vi "Open_WeatherStation_Connection.vi"(1 "Station ID":i32, 2 "Baud rate":i32, 3 "COM port":i32) -> (0 "Weather station connected?":bool)   [LabVIEW 2013]
uses:
  Globals/USB_WeatherLink_Serialnumber.vi
  VantagePro.dll
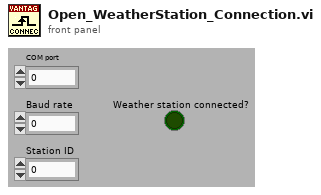
[diagram p1: front panel]
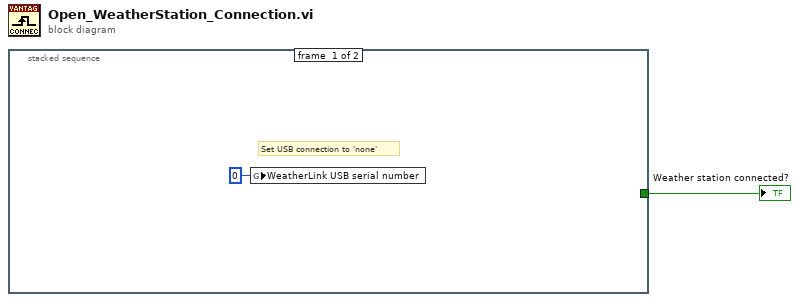
[diagram p0: block diagram]
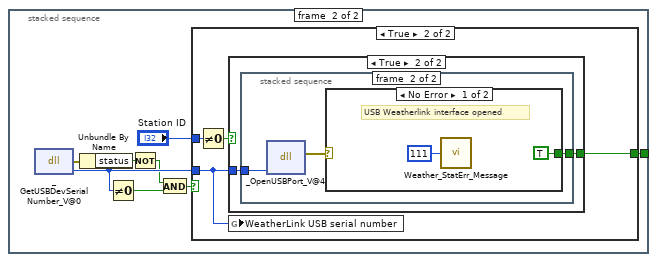
[diagram p2: hidden frame]
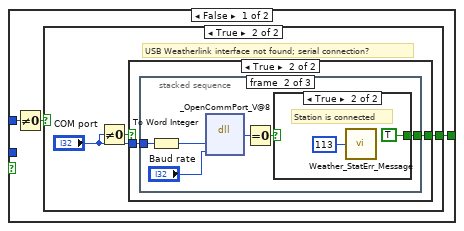
[diagram p3: hidden frame]
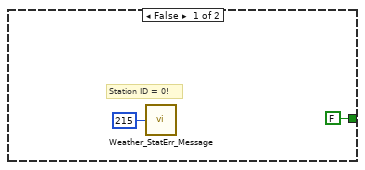
[diagram p4: hidden frame]
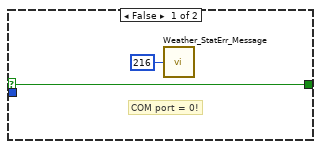
[diagram p5: hidden frame]
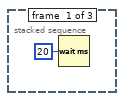
[diagram p6: hidden frame]
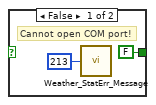
[diagram p7: hidden frame]
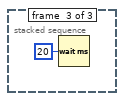
[diagram p8: hidden frame]
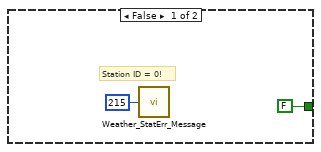
[diagram p9: hidden frame]
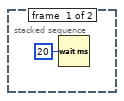
[diagram p10: hidden frame]
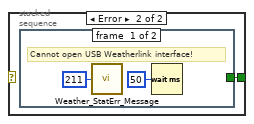
[diagram p11: hidden frame]
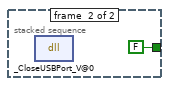
[diagram p12: hidden frame]
diagram:
  n1 = stacked-sequence {
    tunnel: [_ w3] -> w1
    frame #0 {
      # "Set USB connection to 'none'"
      n2 = global write "USB_WeatherLink_Serialnumber.vi" "WeatherLink USB serial number"(u32 0 ("WeatherLink USB serial number")) -> ()
    }
    frame #1 {
      n3 = dll-call lib="C:/Users/Bob van Eijk/Desktop/LabView Projects 13/HiSPARC Weather Station/Develop/VantagePro.dll" fn="_GetUSBDevSerialNumber_V@0" label="Get USB Device\nSerial Number"() -> (error out=w9:errorcluster, "return type"=w8:u32)  [unwired: 3 in, 1 out]
      n4 = Unbundle By Name(w9) -> ("status"=w6:bool)
      n5 = Not Equal To 0?(x=w8) -> (x != 0?=w7:bool)
      n6 = Not(x=w6) -> (.not. x?=w5:bool)
      n7 = And(x=w5, y=w7) -> (x .and. y?=w10:bool)
      n8 = case shown="True" w10 {
        tunnel: [w13 w38] -> w3
        tunnel: w8 -> [_ w35]
        tunnel: "Station ID" -> [w12 w37]
        frame False {
          n9 = Not Equal To 0?(x=w12) -> (x != 0?=w11:bool)
          n10 = case shown="True" w11 {
            tunnel: [FALSE w16] -> w13
            frame False {
              # "Station ID = 0!"
              n11 = call "Weather_StatErr_Message.vi"("Message number"=215) -> ()  [unwired: 1 out]
            }
            frame True {
              # "USB Weatherlink interface not found; serial connection?"
              n12 = Not Equal To 0?(x="COM port") -> (x != 0?=w18:bool)
              n13 = case shown="True" w18 {
                selector: w18 -> [w20 _]
                tunnel: "COM port" -> [_ w22]
                tunnel: [w20 w21] -> w16
                frame False {
                  # "COM port = 0!"
                  n14 = call "Weather_StatErr_Message.vi"("Message number"=216) -> ()  [unwired: 1 out]
                }
                frame True {
                  n15 = stacked-sequence {
                    tunnel: w22 -> [_ w28 _]
                    tunnel: [_ w24 _] -> w21
                    frame #0 {
                      n16 = Wait (ms)(milliseconds to wait=u32 20) -> ()  [unwired: 1 out]
                    }
                    frame #1 {
                      n17 = To Word Integer(number=w28) -> (16bit integer=w27:i16)
                      n18 = dll-call lib="C:/Users/Bob van Eijk/Desktop/LabView Projects 13/HiSPARC Weather Station/Develop/VantagePro.dll" fn="_OpenCommPort_V@8" label="OpenCommPort_V"("comPort"=w27, "baudRate"="Baud rate") -> ("return type"=w26:i16)  [unwired: 4 in, 3 out]
                      n19 = Equal To 0?(x=w26) -> (x = 0?=w25:bool)
                      n20 = case shown="True" w25 {
                        tunnel: [FALSE TRUE] -> w24
                        frame False {
                          # "Cannot open COM port!"
                          n21 = call "Weather_StatErr_Message.vi"("Message number"=213) -> ()  [unwired: 1 out]
                        }
                        frame True {
                          # "Station is connected"
                          n22 = call "Weather_StatErr_Message.vi"("Message number"=113) -> ()  [unwired: 1 out]
                        }
                      }
                    }
                    frame #2 {
                      n23 = Wait (ms)(milliseconds to wait=u32 20) -> ()  [unwired: 1 out]
                    }
                  }
                }
              }
            }
          }
        }
        frame True {
          n24 = Not Equal To 0?(x=w37) -> (x != 0?=w36:bool)
          n25 = case shown="True" w36 {
            tunnel: [FALSE ("USB interface?") w42] -> w38
            tunnel: w35 -> [_ w41]
            frame False {
              # "Station ID = 0!"
              n26 = call "Weather_StatErr_Message.vi"("Message number"=215) -> ()  [unwired: 1 out]
            }
            frame True {
              n27 = stacked-sequence {
                tunnel: [_ w46] -> w42
                tunnel: w41 -> [_ w45]
                frame #0 {
                  n28 = Wait (ms)(milliseconds to wait=u32 20) -> ()  [unwired: 1 out]
                }
                frame #1 {
                  n29 = dll-call lib="C:/Users/Bob van Eijk/Desktop/LabView Projects 13/HiSPARC Weather Station/Develop/VantagePro.dll" fn="_OpenUSBPort_V@4" label="Open USB Port"("USBSerialNumber"=w45) -> (error out=w44:errorcluster)  [unwired: 3 in, 3 out]
                  n30 = case shown="No Error" w44 {
                    tunnel: [TRUE ("USB interface?") w49] -> w46
                    frame No Error {
                      # "USB Weatherlink interface opened"
                      n31 = call "Weather_StatErr_Message.vi"("Message number"=111) -> ()  [unwired: 1 out]
                    }
                    frame Error {
                      n32 = stacked-sequence {
                        tunnel: [_ FALSE ("USB interface?")] -> w49
                        frame #0 {
                          # "Cannot open USB Weatherlink interface!"
                          n33 = call "Weather_StatErr_Message.vi"("Message number"=211) -> ()  [unwired: 1 out]
                          n34 = Wait (ms)(milliseconds to wait=u32 50) -> ()  [unwired: 1 out]
                        }
                        frame #1 {
                          n35 = dll-call lib="C:/Users/Bob van Eijk/Desktop/LabView Projects 13/HiSPARC Weather Station/Develop/VantagePro.dll" fn="_CloseUSBPort_V@0" label="Close USB Port"() -> ()  [unwired: 3 in, 3 out]
                        }
                      }
                    }
                  }
                }
              }
            }
          }
          n36 = global write "USB_WeatherLink_Serialnumber.vi" "WeatherLink USB serial number"(w35) -> ()
        }
      }
    }
  }
  "Weather station connected?" <- w1
